vi "FC Logic.vi"(11 "Log Iteration":i32) -> (2 "Column":i32, 3 "Row":i32)   [LabVIEW 2020]
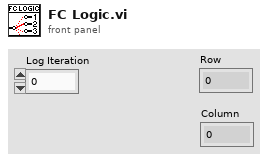
[diagram p1: front panel]
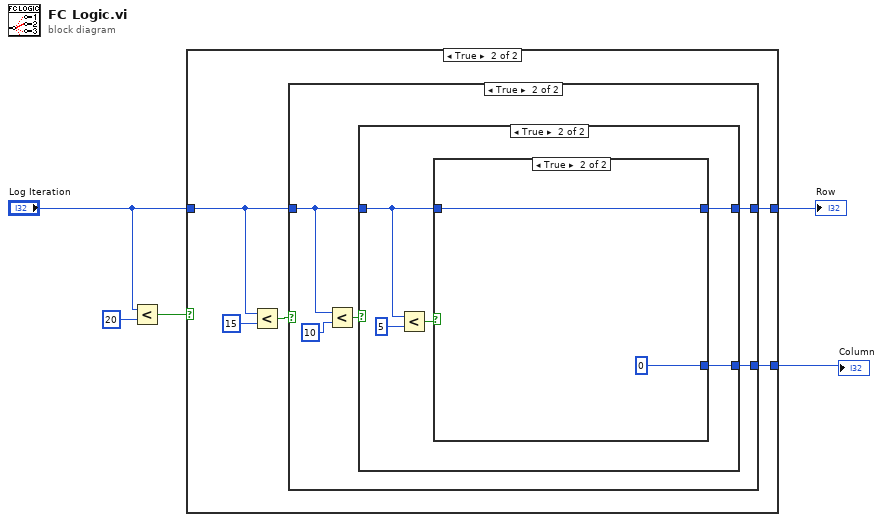
[diagram p0: block diagram]
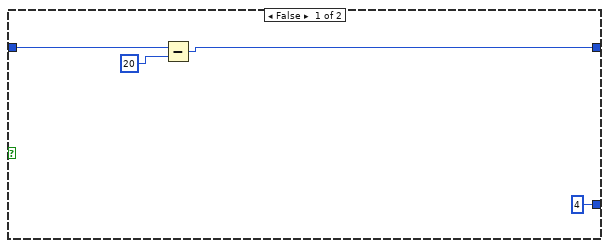
[diagram p2: hidden frame]
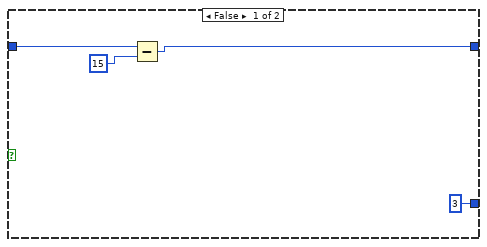
[diagram p3: hidden frame]
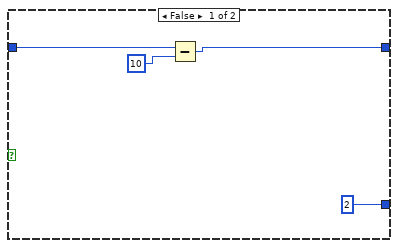
[diagram p4: hidden frame]
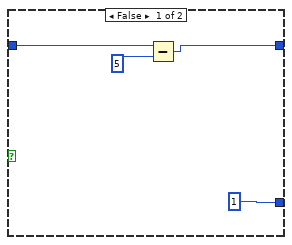
[diagram p5: hidden frame]
diagram:
  n1 = Less?(x="Log Iteration", y=20) -> (x < y?=w4:bool)
  n2 = case shown="True" w4 {
    tunnel: "Log Iteration" -> [w8 w12]
    tunnel: [4 w11] -> w2
    tunnel: [w7 w10] -> w1
    frame False {
      n3 = Subtract(x=w8, y=20) -> (x-y=w7:i32)
    }
    frame True {
      n4 = Less?(x=w12, y=15) -> (x < y?=w13:bool)
      n5 = case shown="True" w13 {
        tunnel: w12 -> [w17 w21]
        tunnel: [3 w20] -> w11
        tunnel: [w16 w19] -> w10
        frame False {
          n6 = Subtract(x=w17, y=15) -> (x-y=w16:i32)
        }
        frame True {
          n7 = Less?(x=w21, y=10) -> (x < y?=w22:bool)
          n8 = case shown="True" w22 {
            tunnel: w21 -> [w26 w29]
            tunnel: [2 w30] -> w20
            tunnel: [w25 w28] -> w19
            frame False {
              n9 = Subtract(x=w26, y=10) -> (x-y=w25:i32)
            }
            frame True {
              n10 = Less?(x=w29, y=5) -> (x < y?=w31:bool)
              n11 = case shown="True" w31 {
                tunnel: [1 0] -> w30
                tunnel: w29 -> [w35 w37]
                tunnel: [w33 w37] -> w28
                frame False {
                  n12 = Subtract(x=w35, y=5) -> (x-y=w33:i32)
                }
                frame True {
                }
              }
            }
          }
        }
      }
    }
  }
  "Column" <- w2
  "Row" <- w1
